vi "Generate 16ms Pulse and ReadACRMSChanValues.vi"(0 "Channel names":string="Dev1/ao3", 1 "nWhichChan":i32, 2 "rate":dbl=10000.0, 3 "frequency":dbl=62.5, 4 "nScale":i32=2, 5 "error in":errorcluster, 8 "offset":dbl=3.75, 9 "SquareWave \nduty cycle (%)":dbl=50.0, 10 "#Samples":i32=1000, 11 "amplitude (pk)":dbl=1.25) -> (14 "task out":refnum<k21>, 15 "Channel Voltage Result":dbl, 19 "error out":errorcluster)   [LabVIEW 2013]
uses:
  <vilib>/DAQmx/write.llb/DAQmx Write (Analog 1D Wfm NChan NSamp).vi
  <vilib>/DAQmx/create/channels.llb/DAQmx Create Channel (AO-Voltage-Basic).vi
  <vilib>/DAQmx/configure/timing.llb/DAQmx Timing (Sample Clock).vi
  <vilib>/DAQmx/miscellaneous.llb/DAQmx Fill In Error Info.vi
  <resource>/objmgr/daqmx.rc
  <vilib>/measure/NI_MABase.lvlib
panel:
  out "Waveform Graph":waveform(dbl)(graph)={"t0"=timestamp(0 s since 1904-01-01), "dt"=0.0001, "Y"=array[1000 elements]}
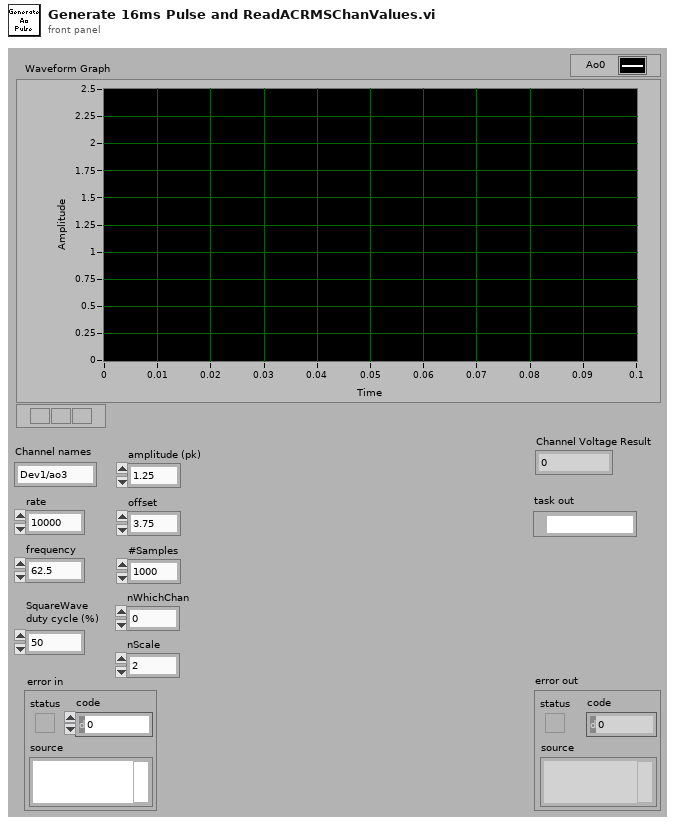
[diagram p1: front panel]
types:
  T1 = enum16{"Sine Wave", "Triangle Wave", "Square Wave", "Sawtooth Wave"}
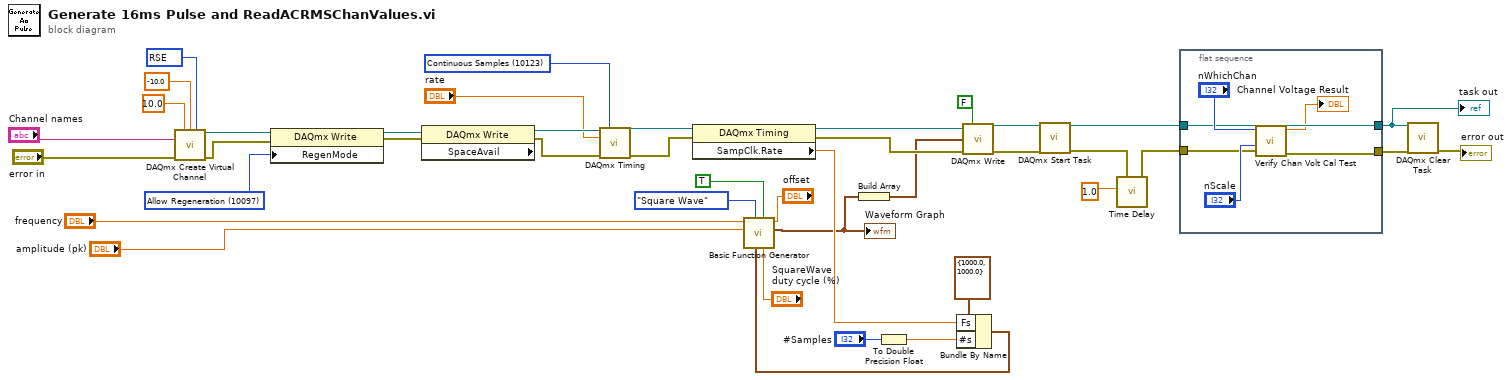
[diagram p0: block diagram]
diagram:
  w8 = 10123 items=["Finite Samples"=10178, "Continuous Samples"=10123, "Hardware Timed Single Point"=12522] ("sample mode")
  w11 = 10083 items=["Default"=-1, "RSE"=10083, "Differential"=10106, "Pseudodifferential"=12529] ("output terminal configuration")
  w39 = 10097 items=["Allow Regeneration"=10097, "Do Not Allow Regeneration"=10158] ("RegenMode")
  n1 = call-poly <vilib>:"DAQmx Create Virtual Channel.vi"("maximum value"=10.0, "minimum value"=-10.0, "output terminal configuration"=w11, "physical channels"="Channel names", "error in"="error in") -> ("task out"=w41:refnum<k21>, "error out"=w40:errorcluster)  [unwired: 9 in]
  n2 = property class="DAQmx Write"(reference=w41, error in=w40, "RegenMode"=w39) -> (reference out=w37:refnum<k21>, error out=w38:errorcluster)
  n3 = property class="DAQmx Write" props=["SpaceAvail"](reference=w37, error in=w38) -> (reference out=w36:refnum<k21>, error out=w35:errorcluster)  [unwired: 1 out]
  n4 = call-poly <vilib>:"DAQmx Timing.vi"("task/channels in"=w36, "sample mode"=w8, "rate"="rate", "error in"=w35) -> ("task out"=w34:refnum<k21>, "error out"=w33:errorcluster)  [unwired: 10 in]
  n5 = property class="DAQmx Timing"(reference=w34, error in=w33) -> (reference out=w16:refnum<k21>, error out=w17:errorcluster, "SampClk.Rate"=w27:dbl)
  n6 = To Double Precision Float(number="#Samples") -> (double precision float=w26:dbl)
  n7 = Bundle By Name(cluster=cluster{"Fs":dbl, "#s":dbl} {"Fs"=1000.0, "#s"=1000.0} ("sampling info"), "Fs"=w27, "#s"=w26) -> (w29:cluster{"Fs":dbl, "#s":dbl})
  n8 = call <vilib>:"Basic Function Generator.vi"("offset"="offset", "square wave duty cycle (%)"="SquareWave \nduty cycle (%)", "reset signal"=TRUE, "sampling info"=w29, "signal type"=T1."Square Wave", "amplitude"="amplitude (pk)", "frequency"="frequency") -> ("signal out"=w9:waveform(dbl))  [unwired: 2 in, 2 out]
  "Waveform Graph" <- w9
  n9 = Build Array(w9) -> (w10:waveform(dbl)[])
  n10 = call-poly <vilib>:"DAQmx Write.vi"("task/channels in"=w16, "auto start"=FALSE, "data"=w10, "error in"=w17) -> ("task out"=w14:refnum<k21>, "error out"=w15:errorcluster)  [unwired: 9 in, 1 out]
  n11 = call <vilib>:"DAQmx Start Task.vi"("task/channels in"=w14, "error in"=w15) -> ("task out"=w6:refnum<k21>, "error out"=w3:errorcluster)  [unwired: 12 in]
  n12 = call "Time Delay"("error in (no error)"=w3, "Delay Time (s)"=1.0) -> ("error out"=w2:errorcluster)  [unwired: 9 in]
  n13 = flat-sequence {
    tunnel: w6 -> [w44]
    tunnel: w2 -> [w43]
    tunnel: [w45] -> w5
    tunnel: [w44] -> w4
    frame #0 {
      n14 = call "Verify Chan Volt Cal Test.vi"("error in (no error)"=w43, "nScale"="nScale", "nWhichChan"="nWhichChan") -> ("error out"=w45:errorcluster, "Channel Voltage Result"=→"Channel Voltage Result":dbl)  [unwired: 7 in]
    }
  }
  n15 = call <vilib>:"DAQmx Clear Task.vi"("task in"=w4, "error in"=w5) -> ("error out"=→"error out":errorcluster)  [unwired: 13 in]
  "task out" <- w4
